vi "Actor Core.vi"(8 "error in":errorcluster, 11 "User Interface in":refnum<class "User Interface.lvclass">) -> (0 "error out":errorcluster, 3 "Actor out":refnum<class "Actor.lvclass">)   [LabVIEW 2020, in "User Interface.lvlib" / "User Interface.lvclass"]
doc: "(<B>Filename</B>: Actor Framework.lvlib:Actor.lvclass:Actor Core.vi)\n\nReceives messages to the actor, reacts to them, and initiates any error handling that may shut the actor down.\n\nDescendant classes may override this VI to append parallel tasks for the actor to complete while it handles messages. Overrides use the Call Parent Class Method node."
uses:
  User Interface.lvclass
  C:/Program Files (x86)/National Instruments/LabVIEW 2020/vi.lib/ActorFramework/Actor/Actor.lvclass
  <vilib>/ActorFramework/Actor/Actor.lvclass
  <vilib>/ActorFramework/Actor/Actor.lvclass/Actor.ctl
  <vilib>/ActorFramework/Message Enqueuer/Message Enqueuer.lvclass/Message Enqueuer.ctl
  User Interface.lvclass/User Interface.ctl
  <vilib>/ActorFramework/Message Enqueuer/Init from Existing Queue.vi
  <vilib>/ActorFramework/Message Enqueuer/Enqueue.vi
  User Interface Messages/Create Sine Wave Msg/Create Sine Wave Msg.lvclass
  C:/Program Files (x86)/National Instruments/LabVIEW 2020/vi.lib/ActorFramework/Message/Message.lvclass
  <vilib>/ActorFramework/Stop Msg/Stop Msg.lvclass
  <vilib>/ActorFramework/Message Priority Queue/Priority Enqueue.vi
  <vilib>/ActorFramework/Message Enqueuer/Message Enqueuer.lvclass
panel:
  in  "stop":bool
  out "Waveform Chart":dbl(graph)
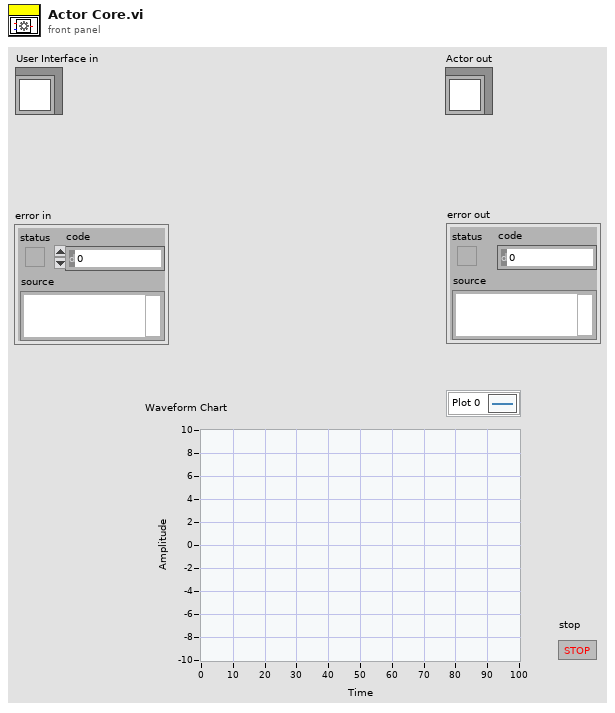
[diagram p1: front panel]
types:
  T1 = enum32{"Invalid", "Standard", "Closed", "Hidden", "Minimized", "Maximized"}
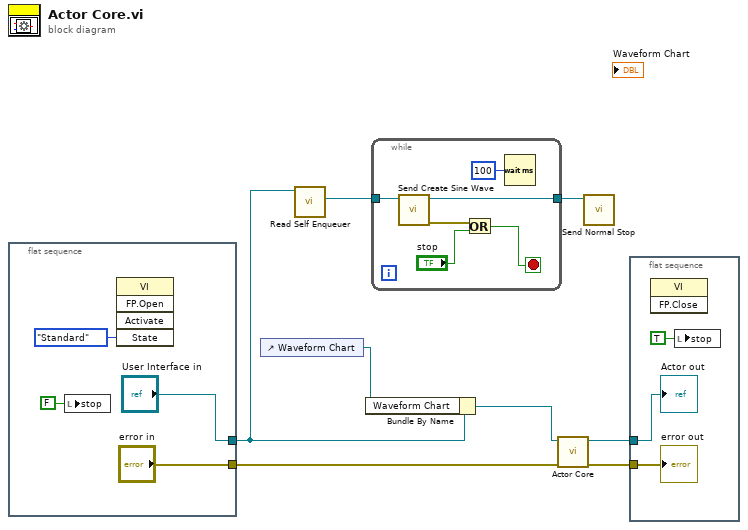
[diagram p0: block diagram]
diagram:
  n1 = flat-sequence {
    tunnel: ["error in"] -> w6
    tunnel: ["User Interface in"] -> w3
    frame #0 {
      n2 = local write "stop"(FALSE ("stop")) -> ()
      n3 = invoke class="VI" method="FP.Open"("State"=T1."Standard") -> ()  [unwired: 4 in, 5 out]
    }
  }
  n4 = control-ref of="Waveform Chart"() -> (w5:refnum<vi>)
  n5 = call <vilib>:"Read Self Enqueuer.vi"("Actor"=w3) -> ("Self Enqueuer"=w2:refnum<class "Message Enqueuer.lvclass">)  [unwired: 10 in]
  n6 = Bundle By Name(cluster=w3, "Waveform Chart"=w5) -> (w4:refnum<class "User Interface.lvclass">)
  n7 = while {
    tunnel: w2 -> [w17]
    tunnel: [w13] -> w1
    stop <- w14 stop-if-true
    n8 = call "Send Create Sine Wave.vi"("Message Enqueuer"=w17) -> ("error out"=w16:errorcluster, "Message Enqueuer out"=w13:refnum<class "Message Enqueuer.lvclass">)  [unwired: 9 in]
    n9 = Or(x=w16, y="stop") -> (x .or. y?=w14:bool)
    n10 = Wait (ms)(milliseconds to wait=u32 100) -> ()  [unwired: 1 out]
  }
  n11 = call-parent "Actor Core.vi"("error in"=w6, "Actor in"=w4) -> ("error out"=w8:errorcluster, "Actor out"=w7:refnum<class "Actor.lvclass">)  [unwired: 8 in]
  n12 = call <vilib>:"Send Normal Stop.vi"("Message Enqueuer"=w1) -> ()  [unwired: 10 in, 1 out]
  n13 = flat-sequence {
    tunnel: w8 -> [w21]
    tunnel: w7 -> [w20]
    frame #0 {
      n14 = invoke class="VI" method="FP.Close"() -> ()  [unwired: 3 in, 3 out]
      n15 = local write "stop"(TRUE ("stop")) -> ()
      "error out" <- w21
      "Actor out" <- w20
    }
  }
